vi "Insert Vi.vi"(7 "Maintain ViValue(F)":bool, 8 "error in (no error)":errorcluster caption="错误输入（无错误）", 9 "ViValue":string, 10 "VI*":refnum<vi>, 11 "PanelDataNode 输入":refnum<class "PanelDataNode.lvclass"> caption="DNL_LabVIEW Object in") -> (0 "error out":errorcluster caption="错误输出", 3 "PanelDataNode 输出":refnum<class "PanelDataNode.lvclass"> caption="DNL_LabVIEW Object out")   [LabVIEW 2016, in "PanelDataNode.lvclass"]
uses:
  PanelDataNode.lvclass
  C:/Users/CL/Desktop/ZcDAQprj0811/ZcDAQprj/Modules/DAQ-Display/PanelSplitToolkit/PanelLinkNode/PanelLinkNode.lvclass
  PanelDataNode.lvclass/PanelDataNode.ctl
  PanelLinkNode/PanelLinkNode.lvclass/PanelLinkNode.ctl
  PanelObject/PanelObject.lvclass
  PanelLinkNode/PanelLinkNode.lvclass
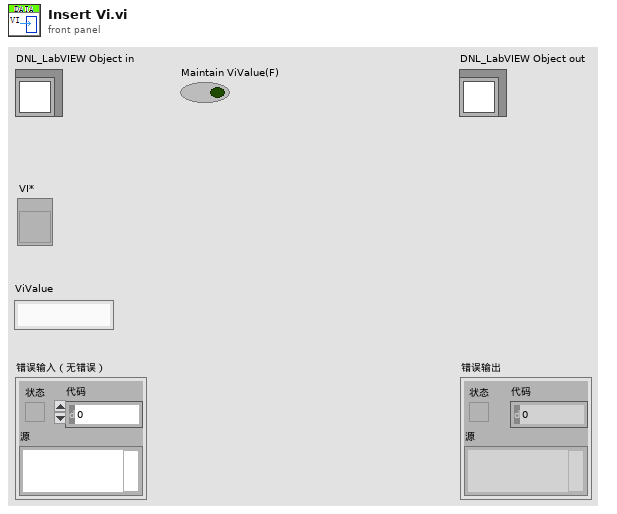
[diagram p1: front panel]
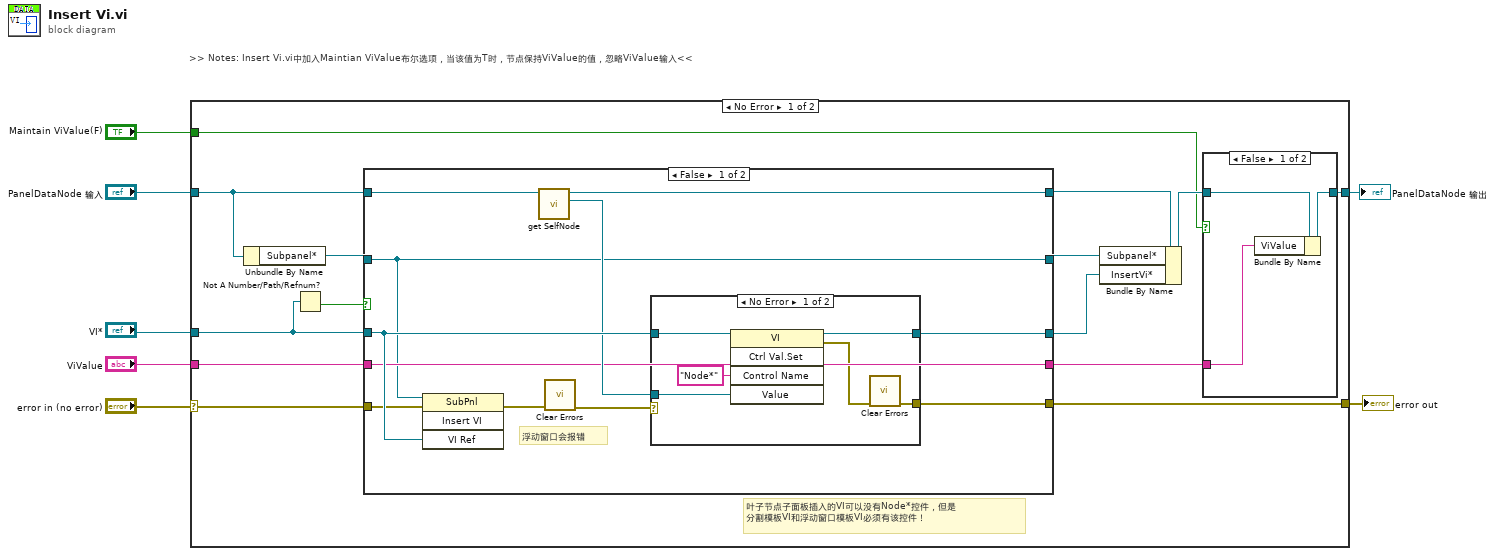
[diagram p0: block diagram]
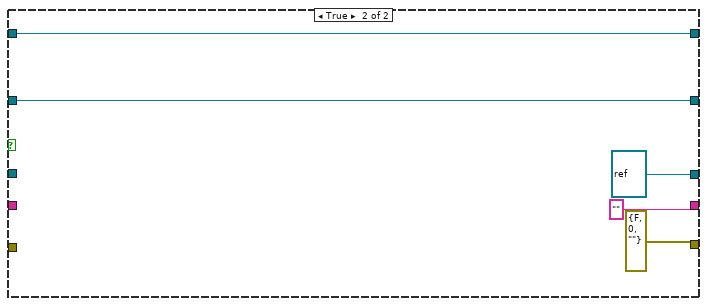
[diagram p4: hidden frame]
diagram:
  # ">> Notes: Insert Vi.vi中加入Maintian ViValue布尔选项，当该值为T时，节点保持ViValue的值，忽略ViValue输入<<"
  n1 = case shown="No Error" "error in (no error)" {
    selector: "error in (no error)" -> [w12 w51]
    tunnel: [w20 w51] -> w6
    tunnel: [w10 w50] -> w4
    tunnel: "PanelDataNode 输入" -> [w16 w50]
    tunnel: "ViValue" -> [w14 _]
    tunnel: "VI*" -> [w13 _]
    tunnel: "Maintain ViValue(F)" -> [w9 _]
    frame No Error {
      # "叶子节点子面板插入的VI可以没有Node*控件，但是\n分割模板VI和浮动窗口模板VI必须有该控件！"
      n2 = Unbundle By Name(w16) -> ("Subpanel*"=w21:refnum<vi>)
      n3 = Not A Number/Path/Refnum?(number/path/refnum=w13) -> (NaN/Path/Refnum?=w18:bool)
      n4 = case shown="False" w18 {
        tunnel: w21 -> [w26 w49]
        tunnel: [w33 errorcluster {"status"=FALSE, "code"=0, "source"=""} ("错误输出")] -> w20
        tunnel: [w26 w49] -> w19
        tunnel: w13 -> [w36 _]
        tunnel: [w35 refnum<vi> refnum ("VI*")] -> w17
        tunnel: w16 -> [w34 w48]
        tunnel: [w32 w48] -> w15
        tunnel: w14 -> [w30 _]
        tunnel: [w30 "" ("ViValue")] -> w8
        tunnel: w12 -> [w27 _]
        frame False {
          # "浮动窗口会报错"
          n5 = invoke class="SubPnl" method="Insert VI"(reference=w26, error in=w27, "VI Ref"=w36) -> (error out=w29:errorcluster)  [unwired: 1 in, 3 out]
          n6 = call "get SelfNode.vi"("PanelLinkNode输入"=w34) -> ("SelfNode*"=w31:refnum<data-value>, "PanelLinkNode输出"=w32:refnum<class "PanelDataNode.lvclass">)  [unwired: 8 in, 1 out]
          n7 = call <vilib>:"Clear Errors.vi"("error in (no error)"=w29) -> ("error out"=w28:errorcluster)  [unwired: 5 in, 1 out]
          n8 = case shown="No Error" w28 {
            selector: w28 -> [_ w44]
            tunnel: w36 -> [w42 w43]
            tunnel: [w41 w43] -> w35
            tunnel: [w38 w44] -> w33
            tunnel: w31 -> [w39 _]
            frame No Error {
              n9 = invoke class="VI" method="Ctrl Val.Set"(reference=w42, "Control Name"="Node*" ("控件名"), "Value"=w39) -> (reference out=w41:refnum<vi>, error out=w37:errorcluster)  [unwired: 2 in, 3 out]
              n10 = call <vilib>:"Clear Errors.vi"("error in (no error)"=w37) -> ("error out"=w38:errorcluster)  [unwired: 5 in, 1 out]
            }
            frame Error {
            }
          }
        }
        frame True {
        }
      }
      n11 = Bundle By Name(cluster=w15, "Subpanel*"=w19, "InsertVi*"=w17) -> (w11:refnum<class "PanelDataNode.lvclass">)
      n12 = case shown="False" w9 {
        tunnel: w11 -> [w24 w25]
        tunnel: [w23 w25] -> w10
        tunnel: w8 -> [w22 _]
        frame False {
          n13 = Bundle By Name(cluster=w24, "ViValue"=w22) -> (w23:refnum<class "PanelDataNode.lvclass">)
        }
        frame True {
        }
      }
    }
    frame Error {
    }
  }
  "error out" <- w6
  "PanelDataNode 输出" <- w4
